vi "Test Write Multiple.vi"(11 "TwinCAT ADS in":refnum<class "TwinCAT ADS.lvclass">) -> (3 "TwinCAT ADS out":refnum<class "TwinCAT ADS.lvclass">)   [LabVIEW 2018]
uses:
  TwinCAT ADS Class/TwinCAT ADS.lvclass
  Controls/Enum.ctl
  Controls/ST_Simple.ctl
  Controls/FB_Complex.ctl
  Controls/ST_Complex.ctl
  Controls/ST_Packed.ctl
  Controls/FB_Simple.ctl
  Controls/FB_Packed.ctl
  e7a7b24b-aede-49d7-b369-bb451e1de87e.vi
  TwinCAT ADS Class/VIs/Data/Read Multiple.vi
  <vilib>/addons/_JKI Toolkits/Caraya/classes/Assert/Assert Equal Value_Variant.vi
  <vilib>/addons/_JKI Toolkits/Caraya/classes/Assert/Assert Equal Value and Type_Variant.vi
  <vilib>/addons/_JKI Toolkits/Caraya/classes/Test/Test.lvclass
  <vilib>/addons/_JKI Toolkits/Caraya/classes/Assert/Assert.lvclass
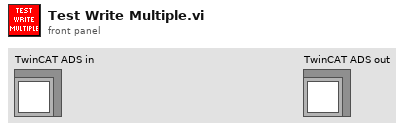
[diagram p1: front panel]
types:
  T1 = typedef "FB_Complex.ctl" = cluster{"_fMember":dbl, "_stMember":T2, "_fbSimpleMember":T6, "_fbPackedMember":T7}
  T2 = typedef "ST_Complex.ctl" = cluster{"bMember":bool, "eMember":T3, "stSimpleMember":T4, "stPackedMember":T5, "FB_Simple":T6, "arrfMember":dbl[]}
  T3 = typedef "Enum.ctl" = enum16{"Member 0", "Member 1", "Member 2"}
  T4 = typedef "ST_Simple.ctl" = cluster{"bMember":bool, "dtMember":timestamp, "nMember":i32}
  T5 = typedef "ST_Packed.ctl" = cluster{"bMember":bool, "dtMember":timestamp, "fMember":dbl}
  T6 = typedef "FB_Simple.ctl" = cluster{"_bMember":bool, "_nMember":i32, "_sMember":string}
  T7 = typedef "FB_Packed.ctl" = cluster{"bMember":bool, "nMember":i32, "sMember":string}
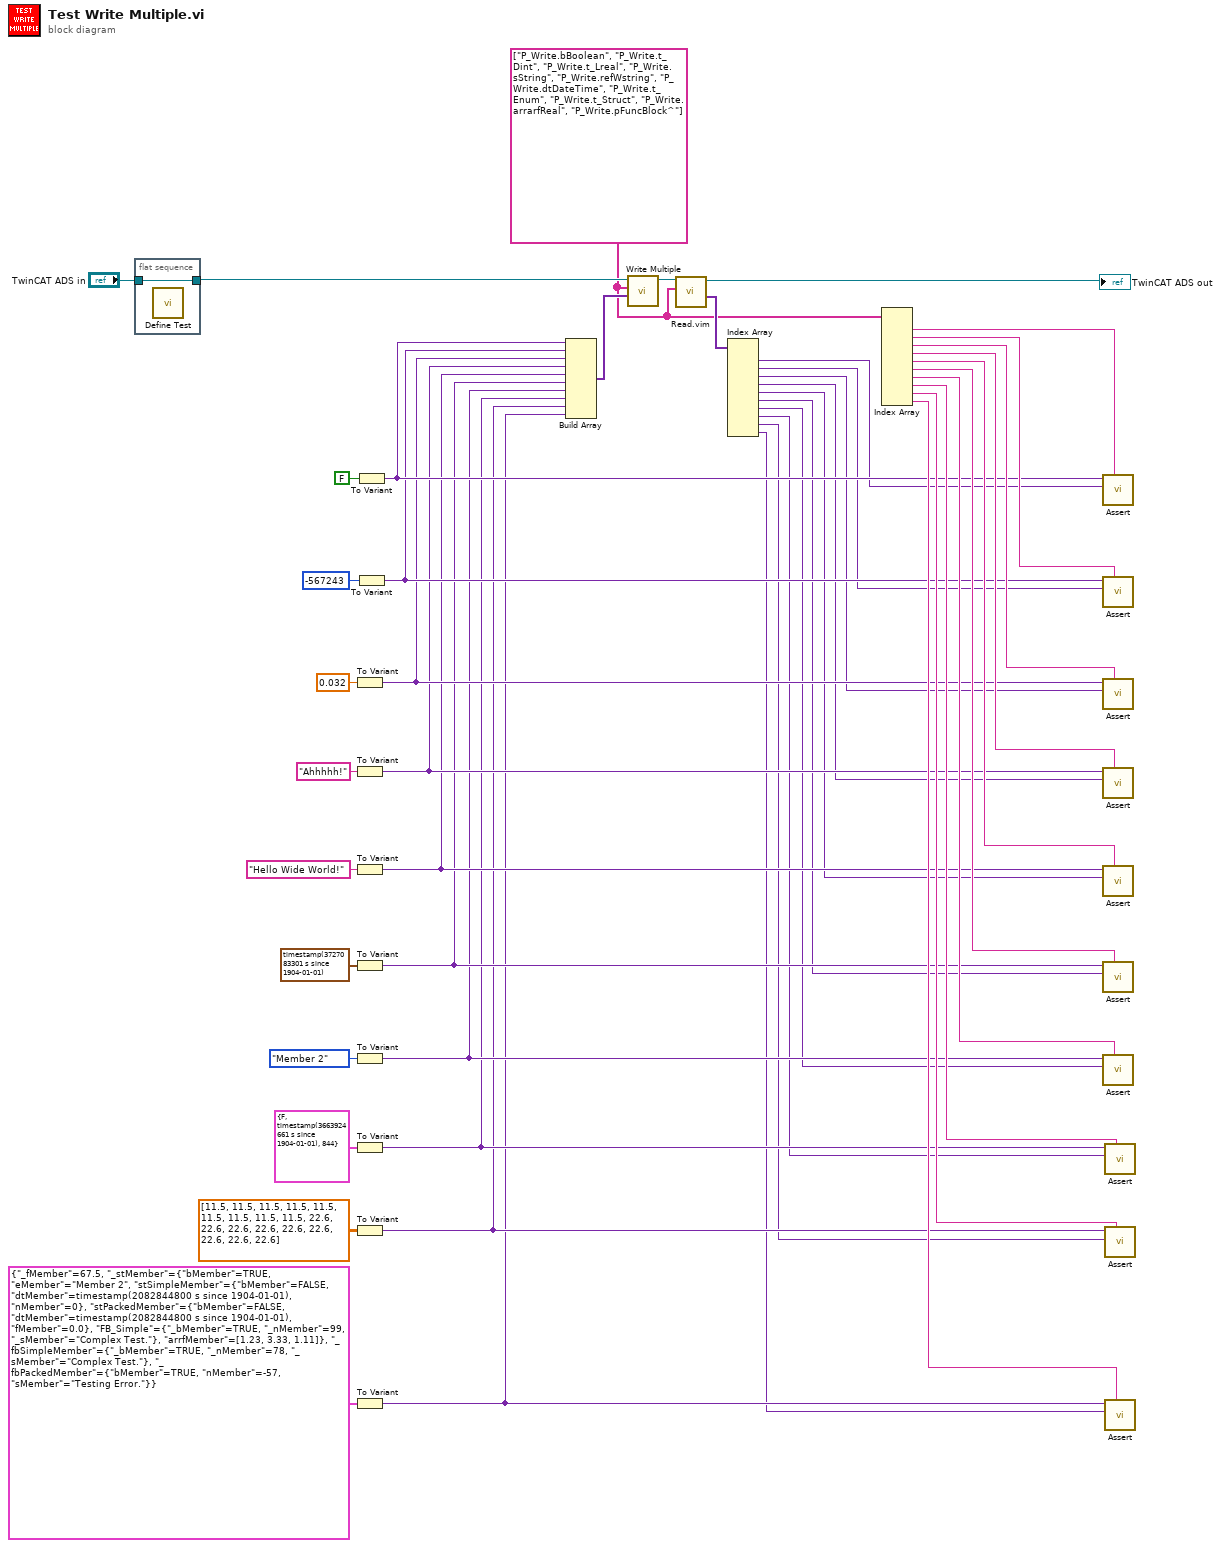
[diagram p0: block diagram]
diagram:
  w1 = string[] ["P_Write.bBoolean", "P_Write.t_Dint", "P_Write.t_Lreal", "P_Write.sString", "P_Write.refWstring", "P_Write.dtDateTime", "P_Write.t_Enum", "P_Write.t_Struct", "P_Write.arrarfReal", "P_Write.pFuncBlock^"]
  n1 = flat-sequence {
    tunnel: "TwinCAT ADS in" -> [w48]
    tunnel: [w48] -> w33
    frame #0 {
      n2 = call <vilib>:"Define Test.vi"() -> ()  [unwired: 10 in, 2 out]
    }
  }
  n3 = To Variant(anything=0.032) -> (Variant=w24:variant)
  n4 = To Variant(anything="Ahhhhh!") -> (Variant=w23:variant)
  n5 = To Variant(anything="Hello Wide World!") -> (Variant=w21:variant)
  n6 = To Variant(anything=timestamp(3727083301 s since 1904-01-01) ("Value")) -> (Variant=w16:variant)
  n7 = To Variant(anything=Enum."Member 2" ("Enum")) -> (Variant=w15:variant)
  n8 = To Variant(anything=T4 {"bMember"=FALSE, "dtMember"=timestamp(3663924661 s since 1904-01-01), "nMember"=844} ("ST_Simple")) -> (Variant=w14:variant)
  n9 = To Variant(anything=dbl[][][] [[[11.5, 11.5, 11.5], [11.5, 11.5, 11.5], [11.5, 11.5, 11.5]], [[22.6, 22.6, 22.6], [22.6, 22.6, 22.6], [22.6, 22.6, 22.6]]]) -> (Variant=w13:variant)
  n10 = To Variant(anything=T1 {"_fMember"=67.5, "_stMember"={"bMember"=TRUE, "eMember"=enum."Member 2", "stSimpleMember"={"bMember"=FALSE, "dtMember"=timestamp(2082844800 s since 1904-01-01), "nMember"=0}, "stPackedMember"={"bMember"=FALSE, "dtMember"=timestamp(2082844800 s since 1904-01-01), "fMember"=0.0}, "FB_Simple"={"_bMember"=TRUE, "_nMember"=99, "_sMember"="Complex Test."}, "arrfMember"=[1.23, 3.33, 1.11]}, "_fbSimpleMember"={"_bMember"=TRUE, "_nMember"=78, "_sMember"="Complex Test."}, "_fbPackedMember"={"bMember"=TRUE, "nMember"=-57, "sMember"="Testing Error."}} ("Value")) -> (Variant=w12:variant)
  n11 = To Variant(anything=FALSE) -> (Variant=w26:variant)
  n12 = To Variant(anything=-567243) -> (Variant=w25:variant)
  n13 = Build Array(w26, w25, w24, w23, w21, w16, w15, w14, w13, w12) -> (w32:variant[])
  n14 = call "Write Multiple.vi"("Values"=w32, "Symbol Names"=w1, "TwinCAT ADS in"=w33) -> ("TwinCAT ADS out"=w34:refnum<class "TwinCAT ADS.lvclass">)  [unwired: 7 in, 1 out]
  n15 = call "Read.vim"("Symbol Name"=w1, "TwinCAT ADS in"=w34) -> ("Value"=w45:variant[], "TwinCAT ADS out"=→"TwinCAT ADS out":refnum<class "TwinCAT ADS.lvclass">)  [unwired: 7 in, 1 out]
  n16 = Index Array(array=w45) -> (element #1=w11:variant, element #2=w10:variant, element #3=w9:variant, element #4=w8:variant, element #5=w7:variant, element #6=w6:variant, element #7=w5:variant, element #8=w4:variant, element #9=w2:variant, element #10=w3:variant)  [unwired: 10 in]
  n17 = Index Array(array=w1) -> (element #1=w44:string, element #2=w43:string, element #3=w42:string, element #4=w41:string, element #5=w40:string, element #6=w39:string, element #7=w38:string, element #8=w37:string, element #9=w36:string, element #10=w35:string)  [unwired: 10 in]
  n18 = call-poly <vilib>:"Assert.vi"("Label"=w44, "Y"=w11, "X"=w26) -> ()  [unwired: 7 in, 2 out]
  n19 = call-poly <vilib>:"Assert.vi"("Label"=w43, "Y"=w10, "X"=w25) -> ()  [unwired: 7 in, 2 out]
  n20 = call-poly <vilib>:"Assert.vi"("Label"=w42, "Y"=w9, "X"=w24) -> ()  [unwired: 7 in, 2 out]
  n21 = call-poly <vilib>:"Assert.vi"("Label"=w41, "Y"=w8, "X"=w23) -> ()  [unwired: 7 in, 2 out]
  n22 = call-poly <vilib>:"Assert.vi"("Label"=w40, "Y"=w7, "X"=w21) -> ()  [unwired: 7 in, 2 out]
  n23 = call-poly <vilib>:"Assert.vi"("Label"=w39, "Y"=w6, "X"=w16) -> ()  [unwired: 7 in, 2 out]
  n24 = call-poly <vilib>:"Assert.vi"("Label"=w38, "Y"=w5, "X"=w15) -> ()  [unwired: 7 in, 2 out]
  n25 = call-poly <vilib>:"Assert.vi"("Label"=w37, "Y"=w4, "X"=w14) -> ()  [unwired: 7 in, 2 out]
  n26 = call-poly <vilib>:"Assert.vi"("Label"=w36, "Y"=w2, "X"=w13) -> ()  [unwired: 7 in, 2 out]
  n27 = call-poly <vilib>:"Assert.vi"("Label"=w35, "Y"=w3, "X"=w12) -> ()  [unwired: 7 in, 2 out]
